vi "LiveAcquisition.vi"() -> ()   [LabVIEW 2018]
uses:
  C:/Users/Dell/Desktop/SIMImaging/Dependencies/PVCamNET.dll
  Dependencies/PVCamNET.dll
panel:
  out "Captured Frames":i64
  in  "?":bool
  in  "?":bool
  in  "Exposure time":u32=5
  # "LiveAcqusition.vi\n\nDescription:\nThis sample code lets the user use live mode \nwith the user's preferred exposure time.\n\nSteps to run:\n1. Click \"Run\"\n2. Enter exposure time\n3. Click \"START\"\n4. Click \"STOP\""
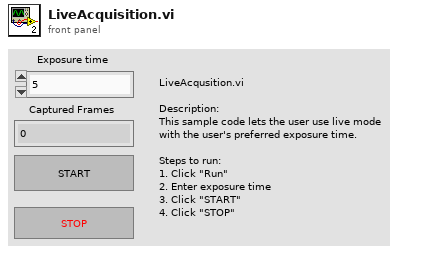
[diagram p1: front panel]
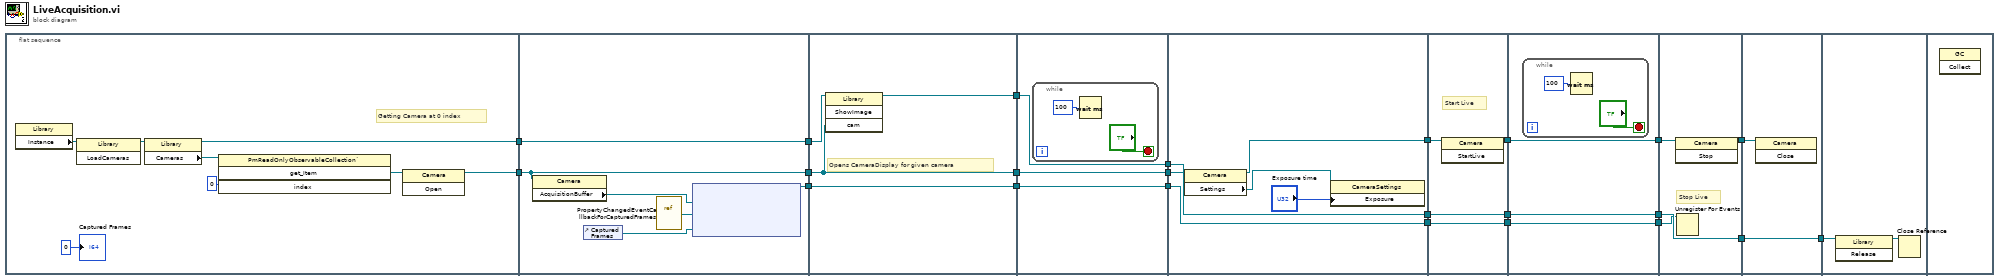
[diagram p0: block diagram]
diagram:
  n1 = flat-sequence {
    tunnel: [w27] -> w11
    tunnel: [w28] -> w9
    tunnel: w11 -> [w37]
    tunnel: [w37] -> w10
    tunnel: w9 -> [w36]
    tunnel: [w36] -> w8
    tunnel: [w32] -> w2
    tunnel: w10 -> [w41]
    tunnel: w8 -> [w40]
    tunnel: [w40] -> w15
    tunnel: [w39] -> w13
    tunnel: [w38] -> w3
    tunnel: w2 -> [w38]
    tunnel: w15 -> [w44]
    tunnel: [w44] -> w14
    tunnel: w13 -> [w43]
    tunnel: [w43] -> w12
    tunnel: [w42] -> w4
    tunnel: w3 -> [w42]
    tunnel: [w52] -> w17
    tunnel: w12 -> [w52]
    tunnel: w14 -> [w51]
    tunnel: [w48] -> w5
    tunnel: w4 -> [w48]
    tunnel: [w47] -> w1
    tunnel: [w55] -> w23
    tunnel: [w54] -> w18
    tunnel: w17 -> [w54]
    tunnel: [w53] -> w6
    tunnel: w5 -> [w53]
    tunnel: w1 -> [w56]
    tunnel: w23 -> [w59]
    tunnel: [w59] -> w22
    tunnel: [w58] -> w19
    tunnel: w18 -> [w58]
    tunnel: [w57] -> w7
    tunnel: w6 -> [w57]
    tunnel: w22 -> [w65]
    tunnel: [w64] -> w21
    tunnel: [w63] -> w20
    tunnel: w19 -> [w63]
    tunnel: w7 -> [w62]
    tunnel: w21 -> [w67]
    tunnel: w20 -> [w66]
    tunnel: [w66] -> w16
    tunnel: w16 -> [w69]
    frame #0 {
      # "Getting Camera at 0 index"
      n2 = property class="Library"() -> ("Instance"=w25:refnum<k24>)  [unwired: 2 in, 2 out]
      n3 = invoke class="Library" method="LoadCameras"(reference=w25) -> (reference out=w24:refnum<k24>)  [unwired: 2 in, 2 out]
      n4 = property class="Library"(reference=w24) -> (reference out=w27:refnum<k24>, "Cameras"=w31:refnum<k24>)  [unwired: 1 in, 1 out]
      n5 = invoke class="PmReadOnlyObservableCollection`" method="get_Item"(reference=w31, "index"=0) -> ("get_Item"=w29:refnum<k24>)  [unwired: 2 in, 3 out]
      n6 = invoke class="Camera" method="Open"(reference=w29) -> (reference out=w28:refnum<k24>)  [unwired: 2 in, 2 out]
      "Captured Frames" <- i64 0 ("Captured (Library counter)")
    }
    frame #1 {
      n7 = property class="Camera"(reference=w36) -> ("AcquisitionBuffer"=w35:refnum<k24>)  [unwired: 1 in, 2 out]
      n8 = control-ref of="Captured Frames"() -> (w34:refnum<vi>)
      n9 = vi-ref "PropertyChangedEventCallbackForCapturedFrames.vi"() -> ("vi reference"=w33:refnum<vi>)
      n10 = node(w35, w33, w34) -> (w32:refnum<k27>)  [unwired: 2 in, 1 out]
    }
    frame #2 {
      # "Opens CameraDisplay for given camera"
      n11 = invoke class="Library" method="ShowImage"(reference=w41, "cam"=w40) -> (reference out=w39:refnum<k24>)  [unwired: 2 in, 3 out]
    }
    frame #3 {
      n12 = while {
        stop <- "?" stop-if-true
        n13 = Wait (ms)(milliseconds to wait=u32 100) -> ()  [unwired: 1 out]
      }
    }
    frame #4 {
      n14 = property class="Camera"(reference=w51) -> (reference out=w47:refnum<k24>, "Settings"=w49:refnum<k24>)  [unwired: 1 in, 1 out]
      n15 = property class="CameraSettings"(reference=w49, "Exposure"="Exposure time") -> ()  [unwired: 1 in, 2 out]
    }
    frame #5 {
      # "Start Live"
      n16 = invoke class="Camera" method="StartLive"(reference=w56) -> (reference out=w55:refnum<k24>)  [unwired: 2 in, 2 out]
    }
    frame #6 {
      n17 = while {
        stop <- "?" stop-if-true
        n18 = Wait (ms)(milliseconds to wait=u32 100) -> ()  [unwired: 1 out]
      }
    }
    frame #7 {
      # "Stop Live"
      n19 = invoke class="Camera" method="Stop"(reference=w65) -> (reference out=w64:refnum<k24>)  [unwired: 2 in, 2 out]
      n20 = Unregister For Events(event registration refnum=w62) -> ()  [unwired: 1 in, 1 out]
    }
    frame #8 {
      n21 = invoke class="Camera" method="Close"(reference=w67) -> ()  [unwired: 2 in, 3 out]
    }
    frame #9 {
      n22 = invoke class="Library" method="Release"(reference=w69) -> (reference out=w68:refnum<k24>)  [unwired: 2 in, 2 out]
      n23 = Close Reference(reference=w68) -> ()  [unwired: 1 in, 1 out]
    }
    frame #10 {
      n24 = invoke class="GC" method="Collect"() -> ()  [unwired: 3 in, 3 out]
    }
  }
